vi "FRIC_navX_Get_Quaternion.vi"(5 "Device Number":T1, 7 "Update":bool) -> (2 "Quaternion":T2)   [LabVIEW 2016]
doc: "This navX VI returns the quaternion of the navX."
uses:
  _TypeDefs/FRIC_navX_DeviceNumbersTypeDef.ctl
  _TypeDefs/Z900_navX_DeviceRegisters.ctl
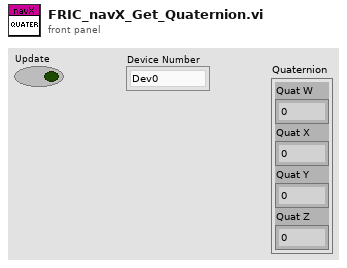
[diagram p1: front panel]
types:
  T1 = typedef "FRIC_navX_DeviceNumbersTypeDef.ctl" = enum16{"Dev0", "Dev1", "Dev2", "Dev3", "Dev4", "Dev5", "Dev6", "Dev7", "Dev8", "Dev9", "Dev10"}
  T2 = cluster{"Quat W":dbl, "Quat X":dbl, "Quat Y":dbl, "Quat Z":dbl}
  T3 = typedef "Z900_navX_DeviceRegisters.ctl" = u8
  T4 = cluster{"Quat W":dbl, "Quat X":dbl, "Quat Y":dbl, "Quat Z":dbl}[]
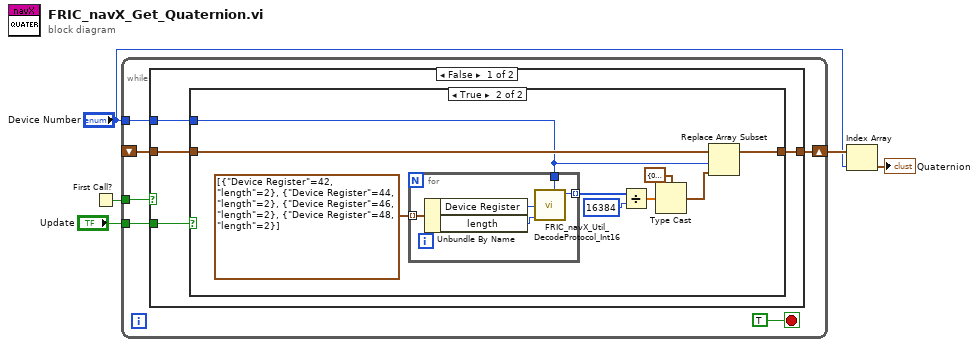
[diagram p0: block diagram]
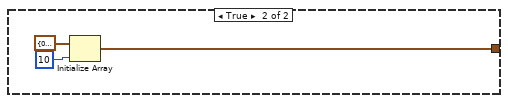
[diagram p3: hidden frame]
diagram:
  n1 = First Call?() -> (First Call?: T/F=w1:bool)
  n2 = while {
    shift-right: [w11] -> w4
    shift-left: _ -> [w10]
    tunnel: "Update" -> [w8]
    tunnel: "Device Number" -> [w7]
    tunnel: w1 -> [w6]
    stop <- TRUE stop-if-true
    n3 = case shown="False" w6 {
      tunnel: [w15 w31] -> w11
      tunnel: w10 -> [w14 _]
      tunnel: w8 -> [w12 _]
      tunnel: w7 -> [w13 _]
      frame False {
        n4 = case shown="True" w12 {
          tunnel: [w16 w19] -> w15
          tunnel: w14 -> [w16 w20]
          tunnel: w13 -> [_ w17]
          frame False {
          }
          frame True {
            n5 = for {
              tunnel: cluster{"Device Register":T3, "length":i32}[] [{"Device Register"=42, "length"=2}, {"Device Register"=44, "length"=2}, {"Device Register"=46, "length"=2}, {"Device Register"=48, "length"=2}] ("Array") -> [w28] mode=indexing
              tunnel: [w27] -> w22 mode=indexing
              tunnel: w17 -> [w26]
              n6 = Unbundle By Name(w28) -> ("Device Register"=w30:T3, "length"=w29:i32)
              n7 = call "FRIC_navX_Util_DecodeProtocol_Int16.vi"("Device Number"=w26, "length"=w29, "Device Register"=w30) -> ("Value"=w27:i16)  [unwired: 8 in]
            }
            n8 = Divide(x=w22, y=u16 16384) -> (x/y=w21:dbl[])
            n9 = Type Cast(type=T2 {"Quat W"=0.0, "Quat X"=0.0, "Quat Y"=0.0, "Quat Z"=0.0}, x=w21) -> (*(type *) &x=w18:T2)
            n10 = Replace Array Subset(array=w20, new element=w18, index=w17) -> (w19:T4)
          }
        }
      }
      frame True {
        n11 = Initialize Array(T2 {"Quat W"=0.0, "Quat X"=0.0, "Quat Y"=0.0, "Quat Z"=0.0}, 10 ("dimension size")) -> (w31:T4)
      }
    }
  }
  n12 = Index Array(array=w4, index="Device Number") -> (element=→"Quaternion":T2)
